vi "conincidences.vi"() -> ()   [LabVIEW 2011]
panel:
  out "Update Count":i32
  out "Penta Coincidences":i32
  in  "Selftest Channel Mask":i32=14
  in  "Exposure Time [ms]":i32=100
  out "Quad Coincidences":i32[](array[numeric])
  out "Triple Coincidences":i32[](array[numeric])
  out "Pair Coincidences":i32[](array[numeric])
  out "Single Counts":i32[](array[numeric])
  out "Error Out":errorcluster
  in  "stop":bool
  in  "Selftest Period [20ns]":i32=10
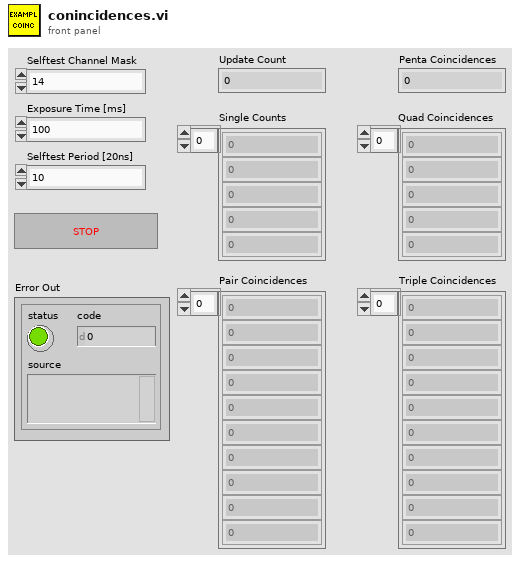
[diagram p1: front panel]
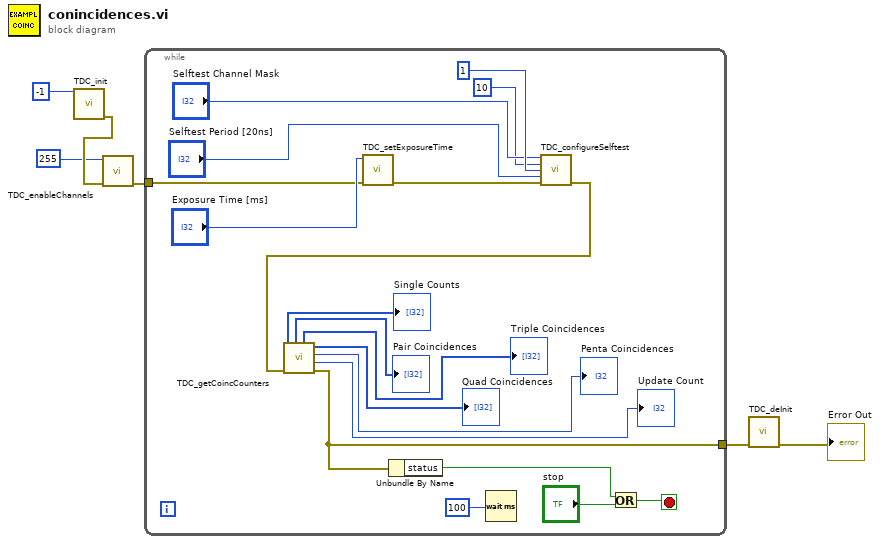
[diagram p0: block diagram]
diagram:
  n1 = call "TDC_init.vi"("Device ID"=-1) -> ("Error Out"=w3:errorcluster)  [unwired: 10 in]
  n2 = call "TDC_enableChannels.vi"("Error In"=w3, "Channel Mask"=255) -> ("Error Out"=w2:errorcluster)  [unwired: 9 in]
  n3 = while {
    tunnel: [w21] -> w5
    tunnel: w2 -> [w9]
    stop <- w25 stop-if-true
    n4 = call "TDC_setExposureTime.vi"("Error In"=w9, "Exposure Time [ms]"="Exposure Time [ms]") -> ("Error Out"=w14:errorcluster)  [unwired: 9 in]
    n5 = Wait (ms)(milliseconds to wait=100) -> ()  [unwired: 1 out]
    n6 = call "TDC_configureSelftest.vi"("Channel Mask"="Selftest Channel Mask", "Period [5ns]"=10, "Burst Size"=1, "Burst Distance [20 ns]"="Selftest Period [20ns]", "Error In"=w14) -> ("Error Out"=w12:errorcluster)  [unwired: 10 in]
    n7 = call "TDC_getCoincCounters.vi"("Error In"=w12) -> ("Error Out"=w21:errorcluster, "Update Count"=→"Update Count":i32, "Penta Coincidences"=→"Penta Coincidences":i32, "Quad Coincidences"=→"Quad Coincidences":i32[], "Triple Coincidences"=→"Triple Coincidences":i32[], "Pair Coincidences"=→"Pair Coincidences":i32[], "Single Counts"=→"Single Counts":i32[])  [unwired: 4 in]
    n8 = Unbundle By Name(w21) -> ("status"=w22:bool)
    n9 = Or(x=w22, y="stop") -> (x .or. y?=w25:bool)
  }
  n10 = call "TDC_deInit.vi"("Error In"=w5) -> ("Error Out"=→"Error Out":errorcluster)  [unwired: 10 in]
